vi "Process Cancel.vi"(6 "Code Previewed?":bool, 8 "error in (no error)":errorcluster, 9 "State Found?":bool, 10 "Preview Visible?":bool, 11 "Queue in":refnum<queue>) -> (0 "error out":errorcluster, 3 "Queue out":refnum<queue>)   [LabVIEW 2021]
uses:
  <vilib>/myRIO/Common/Express VI Framework/typedefs/Config Dlg Actions.ctl
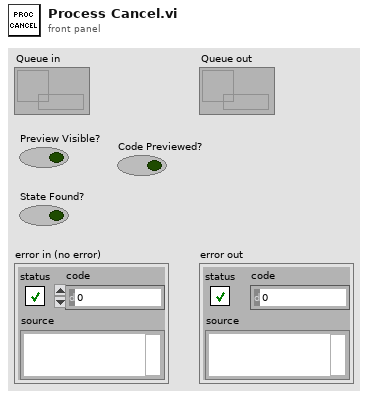
[diagram p1: front panel]
types:
  T1 = typedef "Config Dlg Actions.ctl" = enum16{"Save Changed Name", "Run Pane (from Cancel)", "Initialize Dialog", "Refresh Sensor List", "Load Exp VI State", "Load Sub Pane State", "Display Dialog", "Save Exp VI State", "Save Sub Pane State", "Run Pane", "Stop Pane", "Preview", "Copy Code", "Script Code", "Reinitialize Config Pane", "Close Panel", "Help", "Get Current FPGA Name", "Check IO Resource", "List Connector", "Show Connector", "Valid Data", "Invalid Data", "Stop Pane (from Cancel)"}
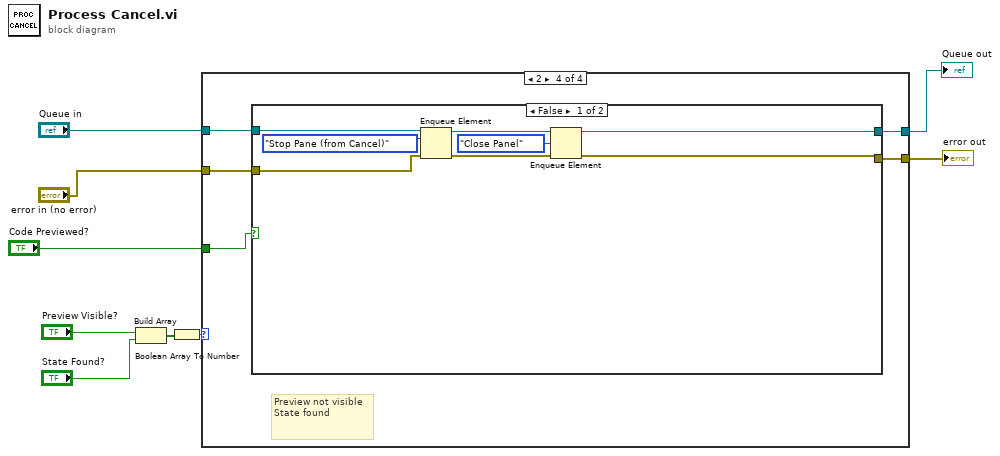
[diagram p0: block diagram]
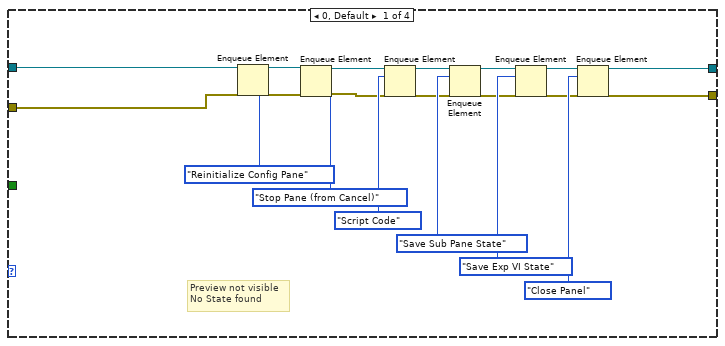
[diagram p2: hidden frame]
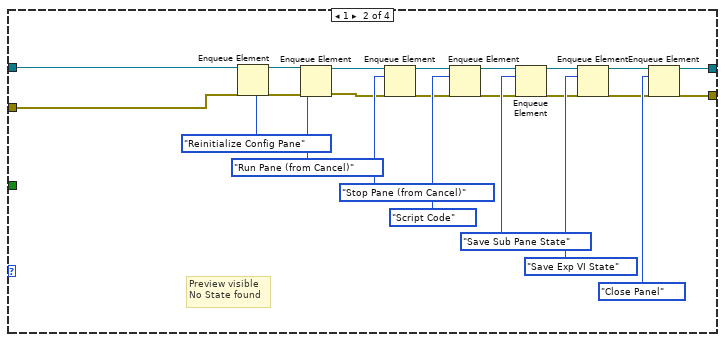
[diagram p3: hidden frame]
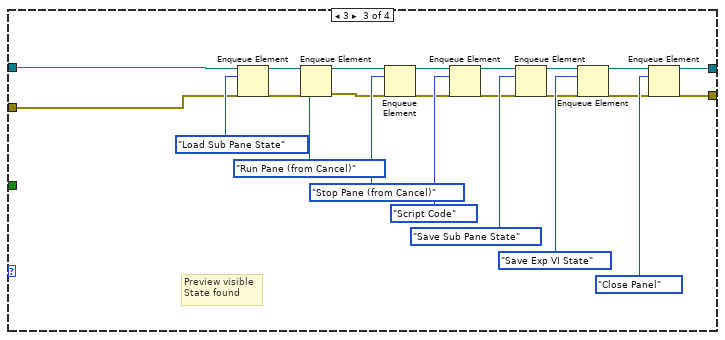
[diagram p4: hidden frame]
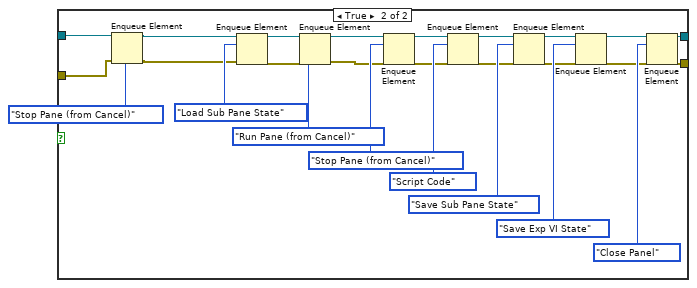
[diagram p5: hidden frame]
diagram:
  n1 = Build Array("Preview Visible?", "State Found?") -> (w4:bool[])
  n2 = Boolean Array To Number(Boolean array=w4) -> (number=w5:u32)
  n3 = case shown="2" w5 {
    tunnel: "error in (no error)" -> [w22 w45 w68 w77]
    tunnel: "Queue in" -> [w23 w46 w69 w78]
    tunnel: [w16 w31 w54 w80] -> w9
    tunnel: [w10 w30 w53 w79] -> w8
    tunnel: "Code Previewed?" -> [_ _ _ w76]
    frame 0, Default {
      # "Preview not visible\nNo State found"
      n4 = Enqueue Element(queue=w23, element=Config_Dlg_Actions."Reinitialize Config Pane" ("Enum"), error in (no error)=w22) -> (queue out=w21:refnum<queue>, error out=w15:errorcluster)  [unwired: 1 in, 1 out]
      n5 = Enqueue Element(queue=w21, element=Config_Dlg_Actions."Stop Pane (from Cancel)" ("Enum"), error in (no error)=w15) -> (queue out=w20:refnum<queue>, error out=w14:errorcluster)  [unwired: 1 in, 1 out]
      n6 = Enqueue Element(queue=w20, element=Config_Dlg_Actions."Script Code" ("Enum"), error in (no error)=w14) -> (queue out=w19:refnum<queue>, error out=w13:errorcluster)  [unwired: 1 in, 1 out]
      n7 = Enqueue Element(queue=w19, element=Config_Dlg_Actions."Save Sub Pane State" ("Enum"), error in (no error)=w13) -> (queue out=w18:refnum<queue>, error out=w12:errorcluster)  [unwired: 1 in, 1 out]
      n8 = Enqueue Element(queue=w18, element=Config_Dlg_Actions."Save Exp VI State" ("Enum"), error in (no error)=w12) -> (queue out=w17:refnum<queue>, error out=w11:errorcluster)  [unwired: 1 in, 1 out]
      n9 = Enqueue Element(queue=w17, element=Config_Dlg_Actions."Close Panel" ("Enum"), error in (no error)=w11) -> (queue out=w10:refnum<queue>, error out=w16:errorcluster)  [unwired: 1 in, 1 out]
    }
    frame 1 {
      # "Preview visible\nNo State found"
      n10 = Enqueue Element(queue=w46, element=Config_Dlg_Actions."Reinitialize Config Pane" ("Enum"), error in (no error)=w45) -> (queue out=w44:refnum<queue>, error out=w37:errorcluster)  [unwired: 1 in, 1 out]
      n11 = Enqueue Element(queue=w44, element=Config_Dlg_Actions."Run Pane (from Cancel)" ("Enum"), error in (no error)=w37) -> (queue out=w43:refnum<queue>, error out=w36:errorcluster)  [unwired: 1 in, 1 out]
      n12 = Enqueue Element(queue=w43, element=Config_Dlg_Actions."Stop Pane (from Cancel)" ("Enum"), error in (no error)=w36) -> (queue out=w42:refnum<queue>, error out=w35:errorcluster)  [unwired: 1 in, 1 out]
      n13 = Enqueue Element(queue=w42, element=Config_Dlg_Actions."Script Code" ("Enum"), error in (no error)=w35) -> (queue out=w41:refnum<queue>, error out=w34:errorcluster)  [unwired: 1 in, 1 out]
      n14 = Enqueue Element(queue=w41, element=Config_Dlg_Actions."Save Sub Pane State" ("Enum"), error in (no error)=w34) -> (queue out=w40:refnum<queue>, error out=w33:errorcluster)  [unwired: 1 in, 1 out]
      n15 = Enqueue Element(queue=w40, element=Config_Dlg_Actions."Save Exp VI State" ("Enum"), error in (no error)=w33) -> (queue out=w39:refnum<queue>, error out=w32:errorcluster)  [unwired: 1 in, 1 out]
      n16 = Enqueue Element(queue=w39, element=Config_Dlg_Actions."Close Panel" ("Enum"), error in (no error)=w32) -> (queue out=w30:refnum<queue>, error out=w31:errorcluster)  [unwired: 1 in, 1 out]
    }
    frame 3 {
      # "Preview visible\nState found"
      n17 = Enqueue Element(queue=w69, element=Config_Dlg_Actions."Load Sub Pane State" ("Enum"), error in (no error)=w68) -> (queue out=w67:refnum<queue>, error out=w60:errorcluster)  [unwired: 1 in, 1 out]
      n18 = Enqueue Element(queue=w67, element=Config_Dlg_Actions."Run Pane (from Cancel)" ("Enum"), error in (no error)=w60) -> (queue out=w66:refnum<queue>, error out=w59:errorcluster)  [unwired: 1 in, 1 out]
      n19 = Enqueue Element(queue=w66, element=Config_Dlg_Actions."Stop Pane (from Cancel)" ("Enum"), error in (no error)=w59) -> (queue out=w65:refnum<queue>, error out=w58:errorcluster)  [unwired: 1 in, 1 out]
      n20 = Enqueue Element(queue=w65, element=Config_Dlg_Actions."Script Code" ("Enum"), error in (no error)=w58) -> (queue out=w64:refnum<queue>, error out=w57:errorcluster)  [unwired: 1 in, 1 out]
      n21 = Enqueue Element(queue=w64, element=Config_Dlg_Actions."Save Sub Pane State" ("Enum"), error in (no error)=w57) -> (queue out=w63:refnum<queue>, error out=w56:errorcluster)  [unwired: 1 in, 1 out]
      n22 = Enqueue Element(queue=w63, element=Config_Dlg_Actions."Save Exp VI State" ("Enum"), error in (no error)=w56) -> (queue out=w62:refnum<queue>, error out=w55:errorcluster)  [unwired: 1 in, 1 out]
      n23 = Enqueue Element(queue=w62, element=Config_Dlg_Actions."Close Panel" ("Enum"), error in (no error)=w55) -> (queue out=w53:refnum<queue>, error out=w54:errorcluster)  [unwired: 1 in, 1 out]
    }
    frame 2 {
      # "Preview not visible\nState found"
      n24 = case shown="False" w76 {
        tunnel: [w83 w95] -> w80
        tunnel: [w86 w94] -> w79
        tunnel: w78 -> [w88 w93]
        tunnel: w77 -> [w85 w92]
        frame False {
          n25 = Enqueue Element(queue=w88, element=Config_Dlg_Actions."Stop Pane (from Cancel)", error in (no error)=w85) -> (queue out=w87:refnum<queue>, error out=w84:errorcluster)  [unwired: 1 in, 1 out]
          n26 = Enqueue Element(queue=w87, element=Config_Dlg_Actions."Close Panel", error in (no error)=w84) -> (queue out=w86:refnum<queue>, error out=w83:errorcluster)  [unwired: 1 in, 1 out]
        }
        frame True {
          n27 = Enqueue Element(queue=w93, element=Config_Dlg_Actions."Stop Pane (from Cancel)", error in (no error)=w92) -> (queue out=w90:refnum<queue>, error out=w89:errorcluster)  [unwired: 1 in, 1 out]
          n28 = Enqueue Element(queue=w90, element=Config_Dlg_Actions."Load Sub Pane State" ("Enum"), error in (no error)=w89) -> (queue out=w108:refnum<queue>, error out=w101:errorcluster)  [unwired: 1 in, 1 out]
          n29 = Enqueue Element(queue=w108, element=Config_Dlg_Actions."Run Pane (from Cancel)" ("Enum"), error in (no error)=w101) -> (queue out=w107:refnum<queue>, error out=w100:errorcluster)  [unwired: 1 in, 1 out]
          n30 = Enqueue Element(queue=w107, element=Config_Dlg_Actions."Stop Pane (from Cancel)" ("Enum"), error in (no error)=w100) -> (queue out=w106:refnum<queue>, error out=w99:errorcluster)  [unwired: 1 in, 1 out]
          n31 = Enqueue Element(queue=w106, element=Config_Dlg_Actions."Script Code" ("Enum"), error in (no error)=w99) -> (queue out=w105:refnum<queue>, error out=w98:errorcluster)  [unwired: 1 in, 1 out]
          n32 = Enqueue Element(queue=w105, element=Config_Dlg_Actions."Save Sub Pane State" ("Enum"), error in (no error)=w98) -> (queue out=w104:refnum<queue>, error out=w97:errorcluster)  [unwired: 1 in, 1 out]
          n33 = Enqueue Element(queue=w104, element=Config_Dlg_Actions."Save Exp VI State" ("Enum"), error in (no error)=w97) -> (queue out=w103:refnum<queue>, error out=w96:errorcluster)  [unwired: 1 in, 1 out]
          n34 = Enqueue Element(queue=w103, element=Config_Dlg_Actions."Close Panel" ("Enum"), error in (no error)=w96) -> (queue out=w94:refnum<queue>, error out=w95:errorcluster)  [unwired: 1 in, 1 out]
        }
      }
    }
  }
  "error out" <- w9
  "Queue out" <- w8
